vi "Project.vi"() -> ()   [LabVIEW 2023]
uses:
  <vilib>/MakerHub/LINX/Public/Peripherals/Analog/Analog Read N Chans.vi
  <vilib>/MakerHub/LINX/Private/Local IO/LinxAnalogRead.vi
  <vilib>/MakerHub/LINX/Public/Utilities/Check Channel.vi
  <vilib>/MakerHub/LINX/Public/Peripherals/PWM/PWM Set Duty Cycle N Chans.vi
  <vilib>/MakerHub/LINX/Private/Utilties/Generate Error.vi
  <vilib>/MakerHub/LINX/Public/Utilities/Open Serial.vi
  <vilib>/addons/control/pid/pid.llb/PID (DBL).vi
  <vilib>/MakerHub/LINX/Public/Peripherals/PWM/PWM Set Duty Cycle 1 Chan.vi
  <vilib>/MakerHub/LINX/Public/Peripherals/Analog/Analog Read 1 Chan.vi
  <vilib>/MakerHub/LINX/LMH-LINX.lvlib
  <vilib>/addons/control/pid/NI_PID_pid.lvlib
panel:
  in  "Enable Heat":bool
  in  "LowPass Filter\nTf = x Ts":dbl
  out "u":dbl format="%_2f V"
  out "Tout":dbl format="%_4f °C"
  in  "Ts":dbl
  out "Waveform Chart":dbl(graph)
  in  "Initial Value":dbl
  in  "Set Point":dbl
  in  "Stop Button":bool
  in  "PID Controller":cluster{"Kp":dbl, "Ti":dbl, "Td":dbl}
  # "Temperature"
  # "Time"
  # "PID Control"
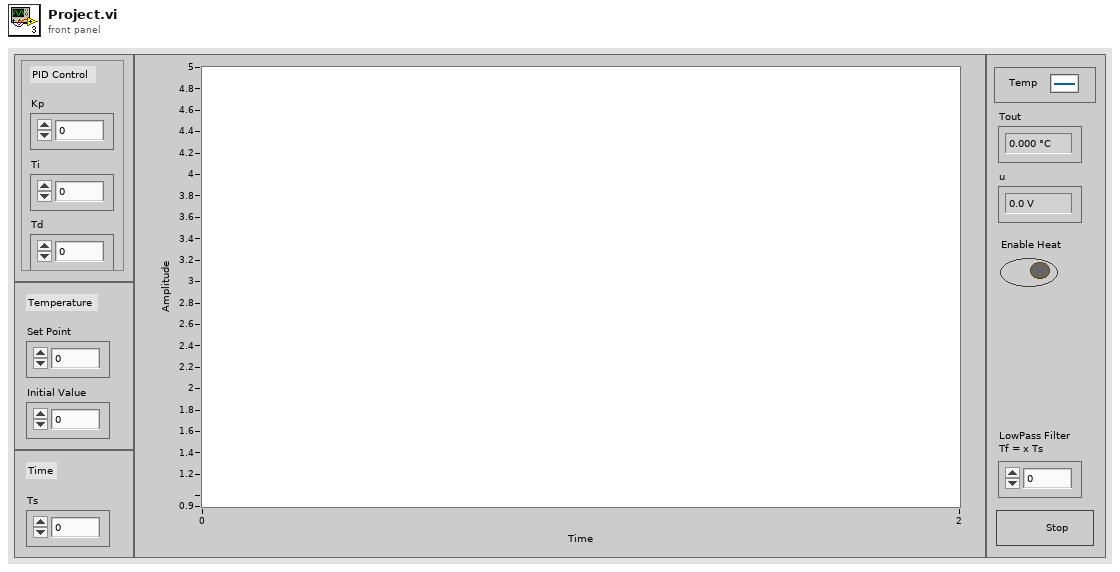
[diagram p1: front panel]
types:
  T1 = typedef "LMH-LINX.lvlib/LINX Ref.ctl" = cluster{"IO":T2, "Interface":T3, "LINX Device Config":T4}
  T2 = typedef "LMH-LINX.lvlib/Platform.ctl" = enum16{"Remote", "Local"}
  T3 = typedef "LMH-LINX.lvlib/Interface.ctl" = enum16{"Serial", "TCP"}
  T4 = typedef "LMH-LINX.lvlib/Device.lvlib/LINX Device Config.ctl" = cluster{"Interface":T3, "COM Port":refnum<visa-resource-name>, "TCP Configuration":T5, "Device Family":u8, "Device ID":u8, "Device Name":string, "TCP Ref":refnum<k5>, "Channels":T6}
  T5 = typedef "LMH-LINX.lvlib/Device.lvlib/TCP Config.ctl" = cluster{"IP Address":string, "Port":u16}
  T6 = typedef "LMH-LINX.lvlib/Channels.ctl" = cluster{"DI":u8[], "DO":u8[], "AI":u8[], "AO":u8[], "PWM":u8[], "QE":u8[], "UART":u8[], "I2C 2":u8[], "SPI":u8[], "CAN":u8[], "Servo":u8[], "AI Ref (V)":dbl, "AI Resolution (Bits)":u8, "AO Ref (V)":dbl, "AO Resolution (Bits)":u8}
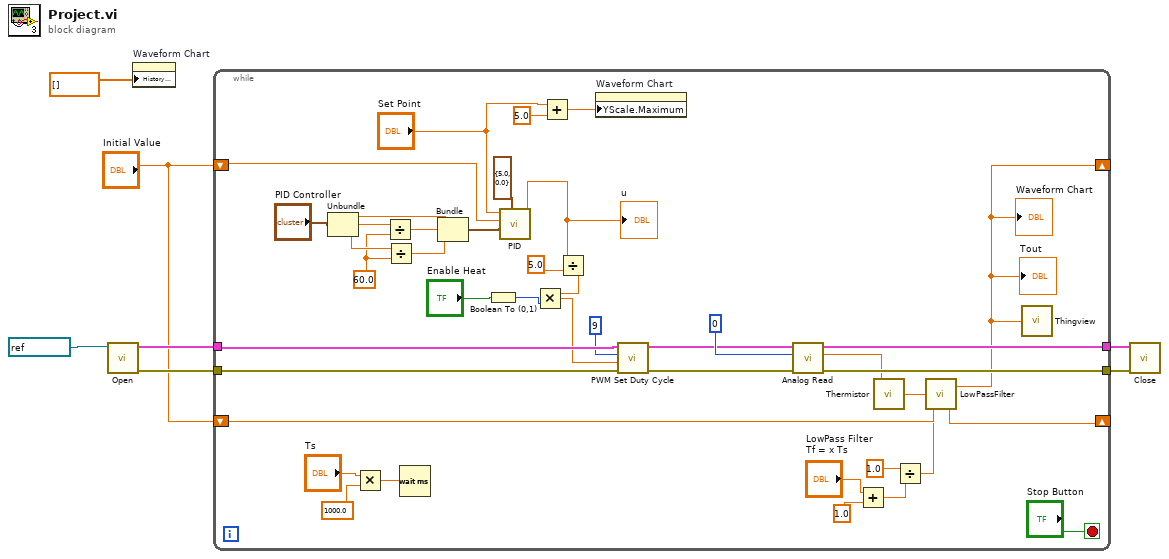
[diagram p0: block diagram]
diagram:
  n1 = call-poly <vilib>:"Open.vi"("Serial Port"=refnum<visa-resource-name> "COM9") -> ("Error Out"=w4:errorcluster, "LINX Resource"=w5:T1)  [unwired: 8 in, 1 out]
  n2 = property on="Waveform Chart" class="WFChart (strict)"("History Data"=dbl[] []) -> ()  [unwired: 2 in, 2 out]
  n3 = while {
    shift-right: [w16] -> _
    shift-left: "Initial Value" -> [w23]
    tunnel: w5 -> [w31]
    tunnel: w4 -> [w29]
    tunnel: [w41] -> w3
    tunnel: [w40] -> w2
    shift-right: [w38] -> _
    shift-left: "Initial Value" -> [w37]
    stop <- "Stop Button" stop-if-true
    w13 = 60.0 ("y")
    n4 = Unbundle("PID Controller") -> ("Kp"=w11:dbl, "Ti"=w15:dbl, "Td"=w14:dbl)
    n5 = Multiply(x="Ts", y=1000.0) -> (x*y=w46:dbl)
    n6 = Divide(x=w15, y=w13) -> (x/y=w12:dbl)
    n7 = Divide(x=w14, y=w13) -> (x/y=w10:dbl)
    n8 = Wait (ms)(milliseconds to wait=w46) -> ()  [unwired: 1 out]
    n9 = Bundle("Kp"=w11, w12, w10) -> (w8:cluster{"Kp":dbl, dbl, dbl})  [unwired: 1 in]
    n10 = Boolean To (0,1)(Boolean="Enable Heat") -> (0, 1=w21:i16)
    n11 = call-poly <vilib>:"PID.vi"("output range"=cluster{"output high":dbl, "output low":dbl} {"output high"=5.0, "output low"=0.0}, "PID gains"=w8, "process variable"=w23, "setpoint"="Set Point") -> ("output"=w19:dbl)  [unwired: 6 in, 1 out]
    "u" <- w19
    n12 = Add(x="Set Point", y=5.0) -> (x+y=w43:dbl)
    n13 = Divide(x=w19, y=5.0) -> (x/y=w18:dbl)
    n14 = Multiply(x=w18, y=w21) -> (x*y=w22:dbl)
    n15 = property on="Waveform Chart" class="WFChart (strict)"("YScale.Maximum"=w43) -> ()  [unwired: 2 in, 2 out]
    n16 = call-poly <vilib>:"PWM Set Duty Cycle.vi"("Error In"=w29, "Duty Cycle (0-1)"=w22, "PWM Channel"=u8 9 ("AO Channel"), "LINX Resource"=w31) -> ("Error Out"=w27:errorcluster, "LINX Resource"=w28:T1)  [unwired: 6 in]
    n17 = call-poly <vilib>:"Analog Read.vi"("Error In"=w27, "Analog Channel"=u8 0, "LINX Resource"=w28) -> ("Error Out"=w40:errorcluster, "Voltage"=w24:dbl, "LINX Resource"=w41:T1)  [unwired: 5 in, 1 out]
    n18 = Add(x="LowPass Filter\nTf = x Ts", y=1.0) -> (x+y=w35:dbl)
    n19 = call "Thermistor.vi"("input variable"=w24) -> ("output variable"=w25:dbl)
    n20 = Divide(x=1.0, y=w35) -> (x/y=w32:dbl)
    n21 = call "LowPassFilter.vi"("a"=w32, "yf_prev"=w37, "Tout"=w25) -> ("yf"=w38:dbl, "Tout"=w16:dbl)
    "Waveform Chart" <- w16
    "Tout" <- w16
    n22 = call "Thingview.vi"("value"=w16) -> ()
  }
  n23 = call <vilib>:"Close.vi"("Error In"=w2, "LINX Resource"=w3) -> ()  [unwired: 9 in, 1 out]
